vi "Read File.vi"(8 "error in (no error)":errorcluster, 11 "Data.TDMS":refnum<class "Data.TDMS.lvclass">) -> (0 "error out":errorcluster, 3 "Data.TDMS out":refnum<class "Data.TDMS.lvclass">)   [LabVIEW 2016, in "Data.TDMS.lvclass"]
uses:
  Data.TDMS.lvclass
  C:/user/patrick/git/LV-to-ITX/src/Data/Data.lvclass
  Data/Data.lvclass/Data.ctl
  Data/Data.lvclass
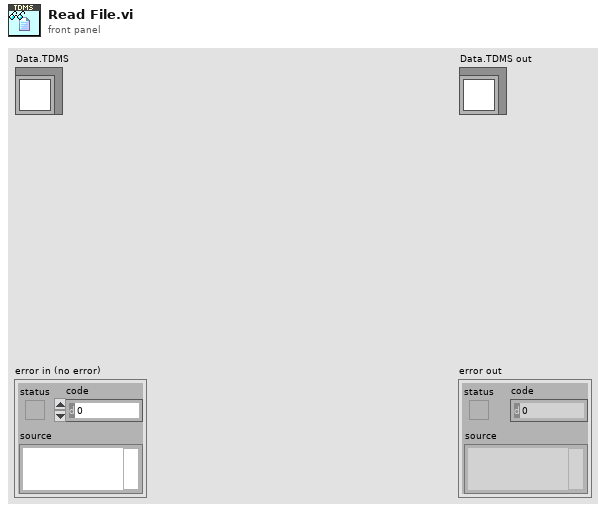
[diagram p1: front panel]
types:
  T1 = typedef "Data.lvclass/Dictionary--cluster.ctl" = cluster{"key":string, "value":variant}
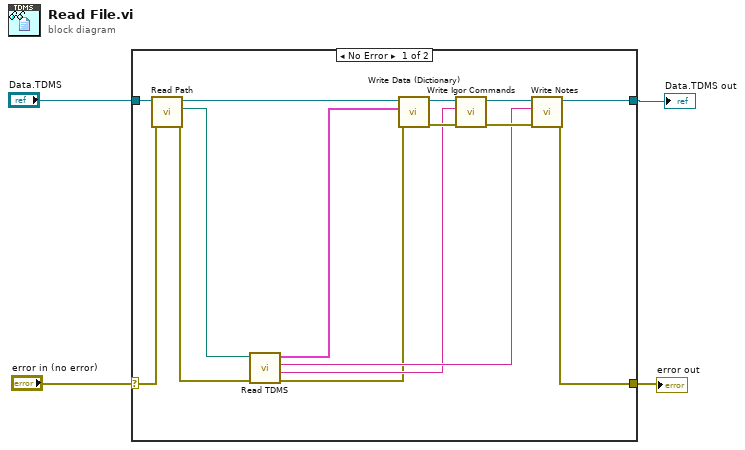
[diagram p0: block diagram]
diagram:
  n1 = case shown="No Error" "error in (no error)" {
    selector: "error in (no error)" -> [w11 w21]
    tunnel: "Data.TDMS" -> [w19 w20]
    tunnel: [w18 w20] -> w2
    tunnel: [w12 w21] -> w1
    frame No Error {
      n2 = call "Read Path.vi"("error in (no error)"=w11, "Data Save"=w19) -> ("error out"=w6:errorcluster, "Path"=w5:path, "Data Save out"=w15:refnum<class "Data.TDMS.lvclass">)  [unwired: 7 in]
      n3 = call "Read TDMS.vi"("error in (no error)"=w6, "path"=w5) -> ("error out"=w7:errorcluster, "Commands"=w8:string, "Notes"=w9:string, "Data (Dictionary)"=w10:T1[])  [unwired: 6 in]
      n4 = call "Write Data (Dictionary).vi"("error in (no error)"=w7, "Data (Dictionary)"=w10, "Data Save"=w15) -> ("error out"=w14:errorcluster, "Data Save out"=w16:refnum<class "Data.TDMS.lvclass">)  [unwired: 7 in]
      n5 = call "Write Igor Commands.vi"("error in (no error)"=w14, "Igor Commands"=w8, "Data Save"=w16) -> ("error out"=w13:errorcluster, "Data Save out"=w17:refnum<class "Data.TDMS.lvclass">)  [unwired: 7 in]
      n6 = call "Write Notes.vi"("error in (no error)"=w13, "Notes"=w9, "Data Save"=w17) -> ("error out"=w12:errorcluster, "Data Save out"=w18:refnum<class "Data.TDMS.lvclass">)  [unwired: 7 in]
    }
    frame Error {
    }
  }
  "error out" <- w1
  "Data.TDMS out" <- w2
